vi "Read_Heater_Channels_fr_File.vi"(1 "Filename":string) -> (0 "Channel Names":string[](array[string]))   [LabVIEW 2022 SP3]
uses:
  Anemometry/Anemometry Sub Vis/Globals/Constants_global.vi
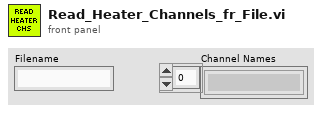
[diagram p1: front panel]
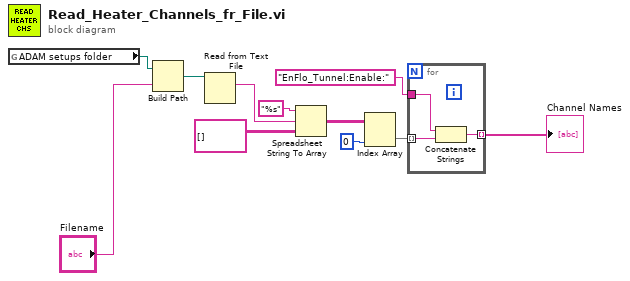
[diagram p0: block diagram]
diagram:
  n1 = global read "Constants_global.vi" "ADAM setups folder"() -> (w6:path)
  n2 = Build Path(base path=w6, name or relative path="Filename") -> (appended path=w2:path)
  n3 = Read from Text File(file (use dialog)=w2) -> (text=w3:string)  [unwired: 3 in, 3 out]
  n4 = Spreadsheet String To Array(format string="%s", spreadsheet string=w3, array type (2D Dbl)=string[][] []) -> (array=w7:string[][])  [unwired: 1 in]
  n5 = Index Array(array=w7, index (col)=0 ("disabled index (col)")) -> (element=w9:string[])  [unwired: 1 in]
  n6 = for {
    tunnel: w9 -> [w14] mode=indexing
    tunnel: [w13] -> w10 mode=indexing
    tunnel: "EnFlo_Tunnel:Enable:" -> [w12]
    n7 = Concatenate Strings(w12, w14) -> (w13:string)
  }
  "Channel Names" <- w10
